vi "Set Available Configurations.vi"(8 "error in (no error)":errorcluster, 11 "Detector Manager in":refnum<class "Detector Manager.lvclass">) -> (0 "error out":errorcluster, 3 "Detector Manager out":refnum<class "Detector Manager.lvclass">)   [LabVIEW 2026, in "TALOS.lvlib" / "Detector Manager.lvlib" / "Detector Manager.lvclass"]
uses:
  Detector Manager.lvclass
  C:/LabVIEW Code/TALOS/talos/Father of all uServices/Father of all uServices/Father of all uServices.lvclass
  Detector Manager.lvclass/Detector Manager.ctl
  Classes/Father of all Detectors/Father Of All Detectors.lvclass
  Father of all uServices/Father of all uServices/Father of all uServices.lvclass
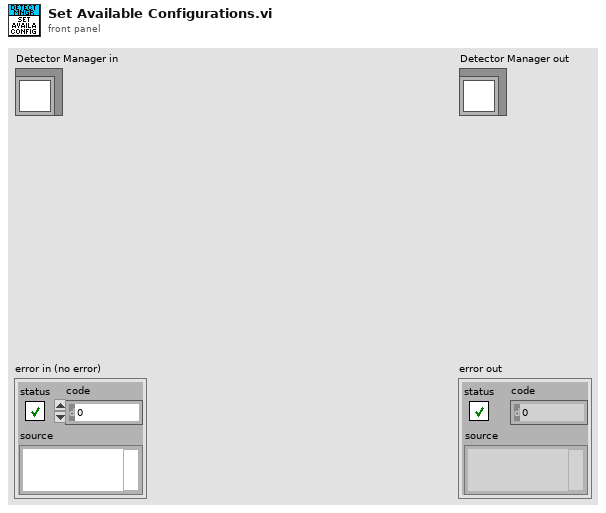
[diagram p1: front panel]
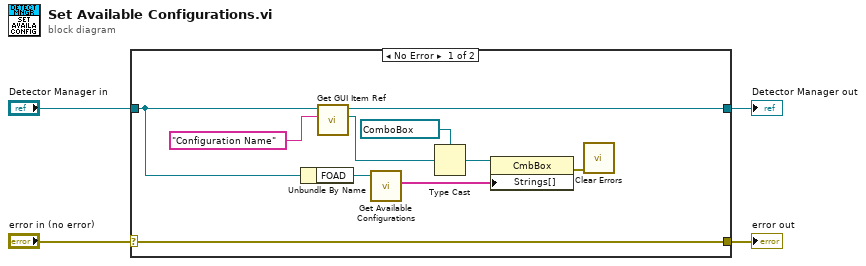
[diagram p0: block diagram]
diagram:
  n1 = case shown="No Error" "error in (no error)" {
    selector: "error in (no error)" -> [w14 w16]
    tunnel: [w14 w16] -> w3
    tunnel: [w10 w15] -> w1
    tunnel: "Detector Manager in" -> [w11 w15]
    frame No Error {
      n2 = Unbundle By Name(w11) -> ("FOAD"=w13:refnum<class "Father Of All Detectors.lvclass">)
      n3 = call "Get GUI Item Ref.vi"("FP Item Name"="Configuration Name", "uService Template in"=w11) -> ("Ctl Refnum"=w9:refnum<vi>, "uService Template out"=w10:refnum<class "Detector Manager.lvclass">)  [unwired: 7 in, 1 out]
      n4 = call-dynamic "Get Available Configurations.vi"("Father Of All Detectors in"=w13) -> ("Configuration names"=w6:string[])  [unwired: 8 in, 2 out]
      n5 = Type Cast(type=refnum<vi> refnum ("CmbBox Refnum"), x=w9) -> (*(type *) &x=w7:refnum<vi>)
      n6 = property class="CmbBox"(reference=w7, "Strings[]"=w6) -> (error out=w5:errorcluster)  [unwired: 1 in, 1 out]
      n7 = call <vilib>:"Clear Errors.vi"("error in (no error)"=w5) -> ()  [unwired: 5 in, 2 out]
    }
    frame Error {
    }
  }
  "error out" <- w3
  "Detector Manager out" <- w1
